vi "Get Charact Standard List.vi"(0 "Path Group in":refnum<class "Path Group.lvclass">, 11 "error in":errorcluster) -> (4 "Path Group out":refnum<class "Path Group.lvclass">, 6 "Charact Standard List":T1[](array[typedef]), 15 "error out":errorcluster)   [LabVIEW 2023, in "RFFixtureCharact.Public.lvlib"]
uses:
  RFFixtureCharact.Public.lvlib
  Common/Base Classes/Path Group/Path Group.lvclass
  Instruments/Cal Standard/Type Definitions/Standard Type.ctl
  Instruments/RFFixtureCharact.Instruments.lvlib
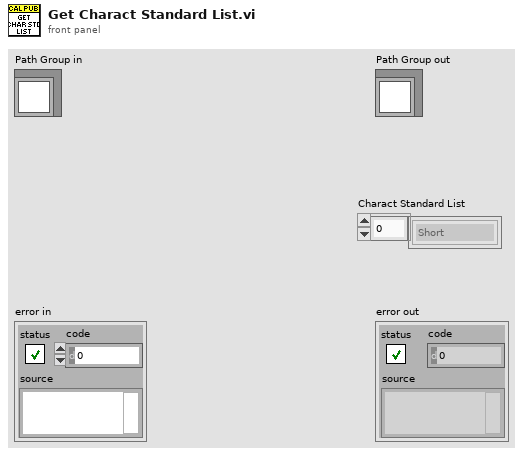
[diagram p1: front panel]
types:
  T1 = typedef "RFFixtureCharact.Instruments.lvlib/Standard Type.ctl" = enum16{"Short", "Open", "Load", "PowerMeter", "None"}
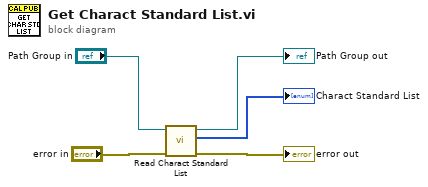
[diagram p0: block diagram]
diagram:
  n1 = call-dynamic "Read Charact Standard List.vi"("error in (no error)"="error in", "Path Group in"="Path Group in") -> ("error out"=→"error out":errorcluster, "Charact Standard List"=→"Charact Standard List":T1[], "Path Group out"=→"Path Group out":refnum<class "Path Group.lvclass">)  [unwired: 7 in]
